vi "Main On Save Action VI.vi"(8 "error in (no error)":errorcluster, 11 "Device Item Ref in":T1 format="%.0x") -> (0 "error out":errorcluster, 3 "Device Item Ref out":T1 format="%.0x")   [LabVIEW 2017, in "Ballard 1553 System Explorer.lvlib"]
uses:
  Ballard 1553 System Explorer.lvlib
  <vilib>/NI Veristand/Custom Device API/Custom Device Item Ref.ctl
  Shared/Controls and Global/Global.vi
  <vilib>/NI Veristand/Custom Device Tools/Custom Device Utility Library/NI VeriStand - Search for All Items by GUID.vi
  <vilib>/NI Veristand/Custom Device API/Get Item Property (I32).vi
  <vilib>/NI Veristand/Custom Device API/Get Item Property (Double).vi
  <userlib>/_OpenG.lib/array/array.llb/Remove Duplicates from 1D Array (U64)__ogtk.vi
  <vilib>/NI Veristand/Custom Device API/Set Item Property (Double).vi
  <vilib>/NI VeriStand/Custom Device API/Custom Device API.lvlib
  <vilib>/NI VeriStand/Custom Device Tools/Custom Device Utility Library/Custom Device Utility Library.lvlib
  Shared/Ballard 1553 Shared.lvlib
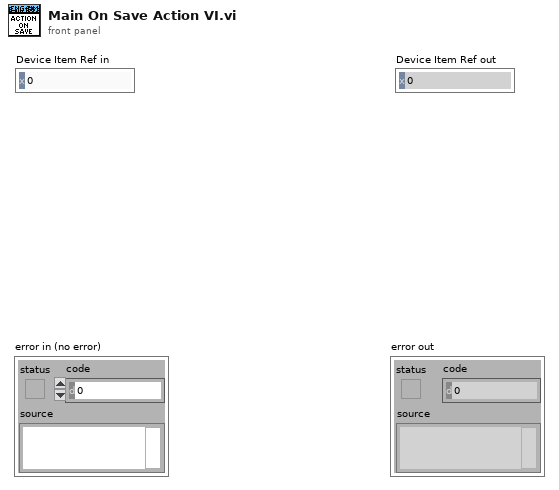
[diagram p1: front panel]
types:
  T1 = typedef "Custom Device API.lvlib/Custom Device Item Ref.ctl" = u64
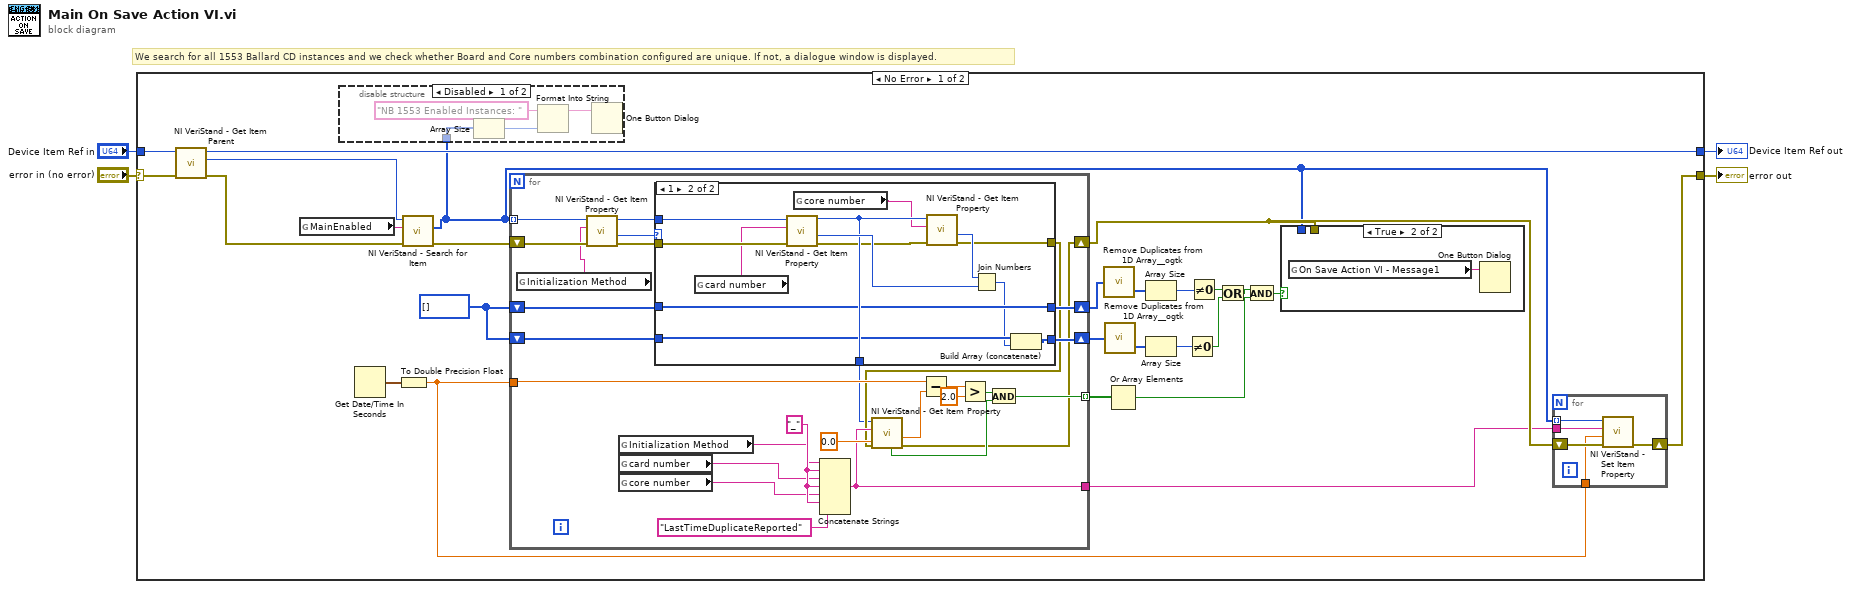
[diagram p0: block diagram]
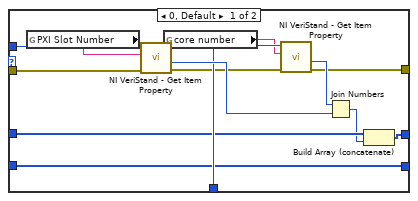
[diagram p4: hidden frame]
diagram:
  # "We search for all 1553 Ballard CD instances and we check whether Board and Core numbers combination configured are unique. If not, a dialogue window is displayed."
  n1 = case shown="No Error" "error in (no error)" {
    selector: "error in (no error)" -> [w30 w95]
    tunnel: [w14 w95] -> w3
    tunnel: "Device Item Ref in" -> [w29 w94]
    tunnel: [w28 w94] -> w1
    frame No Error {
      w13 = u64[] []
      n2 = call <vilib>:"NI VeriStand - Get Item Parent.vi"("error in (no error)"=w30, "Item Ref in"=w29) -> ("error out"=w26:errorcluster, "Parent Ref"=w27:T1, "Item Ref out"=w28:T1)  [unwired: 6 in, 1 out]
      n3 = global read "Global.vi" "MainEnabled"() -> (w5:string)
      n4 = Get Date/Time In Seconds() -> (seconds since 1Jan1904=w22:timestamp)
      n5 = To Double Precision Float(number=w22) -> (double precision float=w19:dbl)
      n6 = call-poly <vilib>:"NI VeriStand - Search for Item.vi"("error in"=w26, "Item GUID"=w5, "Section Ref in"=w27) -> ("error out"=w25:errorcluster, "Item Refs"=w21:T1[])  [unwired: 5 in, 2 out]
      n7 = disable-structure shown="Disabled" {
        disable-tunnel: w21 -> [w39 _]
        frame Disabled {
          n8 = Array Size(array=w39) -> (size(s)=w38:i32)
          n9 = Format Into String(initial string="NB 1553 Enabled Instances: ", w38) -> (resulting string=w37:string)  [unwired: 2 in, 1 out]
          n10 = One Button Dialog(message=w37) -> ()  [unwired: 1 in, 1 out]
        }
        frame Enabled {
        }
      }
      n11 = for {
        tunnel: w21 -> [w57] mode=indexing
        shift-right: [w46] -> w23
        shift-left: w25 -> [w55]
        tunnel: w19 -> [w66]
        tunnel: [w60] -> w16 mode=indexing
        tunnel: [w59] -> w20
        shift-right: [w51] -> w12
        shift-left: w13 -> [w52]
        shift-right: [w49] -> w11
        shift-left: w13 -> [w50]
        w48 = "_"
        n12 = global read "Global.vi" "Initialization Method"() -> (w44:string)
        n13 = call-poly <vilib>:"NI VeriStand - Get Item Property.vi"("error in (no error)"=w55, "Property Name"=w44, "Item Ref in"=w57) -> ("error out"=w54:errorcluster, "Value"=w53:i32, "Item Ref out"=w56:T1)  [unwired: 5 in, 1 out]
        n14 = global read "Global.vi" "Initialization Method"() -> (w43:string)
        n15 = global read "Global.vi" "card number"() -> (w42:string)
        n16 = global read "Global.vi" "core number"() -> (w41:string)
        n17 = case shown="1" w53 {
          tunnel: [w78 w91] -> w47
          tunnel: [w77 w90] -> w45
          tunnel: w56 -> [w76 w89]
          tunnel: w54 -> [w75 w88]
          tunnel: w52 -> [w74 w87]
          tunnel: [w73 w87] -> w51
          tunnel: w50 -> [w72 w86]
          tunnel: [w72 w85] -> w49
          frame 0, Default {
            n18 = global read "Global.vi" "PXI Slot Number"() -> (w69:string)
            n19 = call-poly <vilib>:"NI VeriStand - Get Item Property.vi"("error in (no error)"=w75, "Property Name"=w69, "Item Ref in"=w76) -> ("error out"=w70:errorcluster, "Value"=w80:i32, "Item Ref out"=w77:T1)  [unwired: 5 in, 1 out]
            n20 = global read "Global.vi" "core number"() -> (w68:string)
            n21 = call-poly <vilib>:"NI VeriStand - Get Item Property.vi"("error in (no error)"=w70, "Property Name"=w68, "Item Ref in"=w77) -> ("error out"=w78:errorcluster, "Value"=w79:i32)  [unwired: 5 in, 2 out]
            n22 = Join Numbers(hi=w79, lo=w80) -> ((hi.lo)=w71:u64)
            n23 = Build Array (concatenate)(w74, w71) -> (w73:u64[])
          }
          frame 1 {
            n24 = global read "Global.vi" "card number"() -> (w82:string)
            n25 = call-poly <vilib>:"NI VeriStand - Get Item Property.vi"("error in (no error)"=w88, "Property Name"=w82, "Item Ref in"=w89) -> ("error out"=w83:errorcluster, "Value"=w93:i32, "Item Ref out"=w90:T1)  [unwired: 5 in, 1 out]
            n26 = global read "Global.vi" "core number"() -> (w81:string)
            n27 = call-poly <vilib>:"NI VeriStand - Get Item Property.vi"("error in (no error)"=w83, "Property Name"=w81, "Item Ref in"=w90) -> ("error out"=w91:errorcluster, "Value"=w92:i32)  [unwired: 5 in, 2 out]
            n28 = Join Numbers(hi=w92, lo=w93) -> ((hi.lo)=w84:u64)
            n29 = Build Array (concatenate)(w86, w84) -> (w85:u64[])
          }
        }
        n30 = Concatenate Strings(w43, w48, w42, w48, w41, w48, "LastTimeDuplicateReported") -> (w59:string)
        n31 = call-poly <vilib>:"NI VeriStand - Get Item Property.vi"("error in (no error)"=w47, "Default Value"=0.0, "Property Name"=w59, "Item Ref in"=w45) -> ("error out"=w46:errorcluster, "Value"=w65:dbl, "Found?"=w61:bool)  [unwired: 4 in, 1 out]
        n32 = Subtract(x=w66, y=w65) -> (x-y=w63:dbl)
        n33 = Greater?(x=w63, y=2.0) -> (0:w62:bool)
        n34 = And(x=w62, y=w61) -> (x .and. y?=w60:bool)
      }
      n35 = call-poly <userlib>:"Remove Duplicates from 1D Array__ogtk.vi"("Input Array"=w12) -> ("indices of removed elements"=w24:i32[])  [unwired: 1 out]
      n36 = call-poly <userlib>:"Remove Duplicates from 1D Array__ogtk.vi"("Input Array"=w11) -> ("indices of removed elements"=w10:i32[])  [unwired: 1 out]
      n37 = Or Array Elements(Boolean array=w16) -> (logical OR=w15:bool)
      n38 = Array Size(array=w24) -> (size(s)=w17:i32)
      n39 = Array Size(array=w10) -> (size(s)=w9:i32)
      n40 = Not Equal To 0?(x=w9) -> (x != 0?=w7:bool)
      n41 = Not Equal To 0?(x=w17) -> (x != 0?=w8:bool)
      n42 = Or(x=w8, y=w7) -> (x .or. y?=w6:bool)
      n43 = And(x=w6, y=w15) -> (x .and. y?=w18:bool)
      n44 = case shown="True" w18 {
        tunnel: w23 -> [_ _]
        tunnel: w21 -> [_ _]
        frame False {
        }
        frame True {
          n45 = global read "Global.vi" "On Save Action VI - Message1"() -> (w40:string)
          n46 = One Button Dialog(message=w40) -> ()  [unwired: 1 in, 1 out]
        }
      }
      n47 = for {
        shift-right: [w34] -> w14
        shift-left: w23 -> [w35]
        tunnel: w21 -> [w33] mode=indexing
        tunnel: w20 -> [w32]
        tunnel: w19 -> [w31]
        n48 = call-poly <vilib>:"NI VeriStand - Set Item Property.vi"("error in (no error)"=w35, "Value"=w31, "Property Name"=w32, "Item Ref in"=w33) -> ("error out"=w34:errorcluster)  [unwired: 5 in, 2 out]
      }
    }
    frame Error {
    }
  }
  "error out" <- w3
  "Device Item Ref out" <- w1
